vi "getDetails.vi"(8 "error in (no error)":errorcluster, 11 "reference in":refnum<class "trackingNotification.lvclass">) -> (0 "error out":errorcluster, 1 "index_parts_expired":i32[](array[numeric]), 2 "data":string[][](array[string]), 3 "reference out":refnum<class "trackingNotification.lvclass">)   [LabVIEW 2014, in "trackingNotification.lvclass"]
uses:
  trackingNotification.lvclass
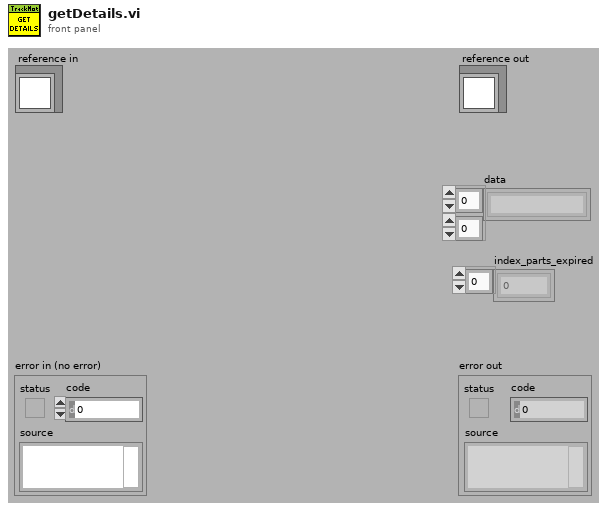
[diagram p1: front panel]
types:
  T1 = typedef "trackingNotification.lvclass/ObjectAttributesRef.ctl" = refnum<data-value>
  T2 = typedef "trackingNotification.lvclass/ObjectAttributes.ctl" = cluster{"MyAttribute":dbl, "index_parts_expired":i32[], "data":string[][]}
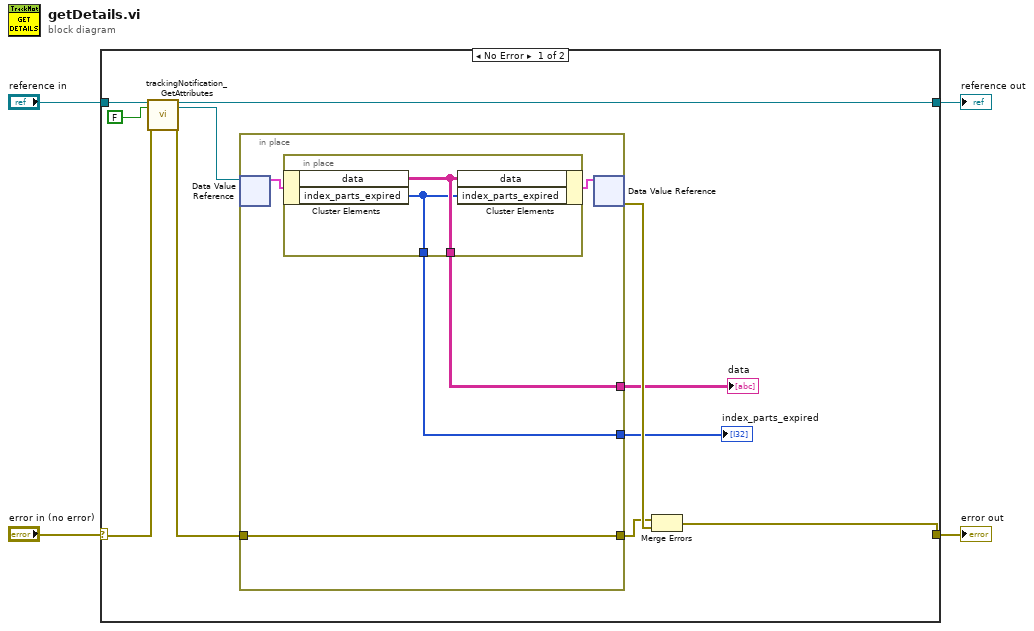
[diagram p0: block diagram]
diagram:
  n1 = case shown="No Error" "error in (no error)" {
    selector: "error in (no error)" -> [w10 w24]
    tunnel: [w15 w24] -> w3
    tunnel: [w8 w23] -> w1
    tunnel: "reference in" -> [w12 w23]
    frame No Error {
      n2 = call "trackingNotification_GetAttributes.vi"("reference in"=w12, "return data? (T)"=FALSE, "error in (no error)"=w10) -> ("reference out"=w8:refnum<class "trackingNotification.lvclass">, "attributes ref"=w7:T1, "error out"=w9:errorcluster)  [unwired: 13 in, 1 out]
      n3 = in-place {
        in-place-border: w9 -> [w18]
        in-place-border: [w18] -> w13
        in-place-border: [w17] -> w6
        in-place-border: [w16] -> w5
        n4 = in-place-dvr #1(w7) -> (w19:T2)  [unwired: 1 out]
        n5 = in-place {
          in-place-border: [w22] -> w17
          in-place-border: [w21] -> w16
          n6 = in-place-cluster #2(w19) -> ("data"=w22:string[][], "index_parts_expired"=w21:i32[])
          n7 = in-place-cluster #2("data"=w22, "index_parts_expired"=w21) -> (w20:T2)
        }
        n8 = in-place-dvr #1(w20) -> (w14:errorcluster)  [unwired: 1 out]
      }
      "data" <- w6
      "index_parts_expired" <- w5
      n9 = Merge Errors(w13, w14) -> (w15:errorcluster)
    }
    frame Error {
    }
  }
  "error out" <- w3
  "reference out" <- w1
